vi "Write String Table.vi"(0 "Report Ref In":T1, 1 "Start Row Index":i32, 2 "Start Column Index":i32, 3 "error in (no error)":errorcluster, 4 "Input Range":string[][](array[string])) -> (5 "Report Ref Out":T1, 6 "error out":errorcluster)   [LabVIEW 2013, in "XCel Report Engine.lvlib"]
doc: "Writes a two-dimensional string array to a rectangular range in the active worksheet.\n\nThe top-left destination cell is specified by zero-based row and column coordinates. Coordinate (0, 0) corresponds to cell A1.\n\nThe number of rows and columns is derived from the dimensions of the input array. Values are written in row-major order, and empty strings create empty string cells.\n\nExisting cell values or formulas in the destination range are replaced while the existing formatting of each cell is preserved. The destination range must remain within the Excel worksheet limits."
uses:
  XCel Report Engine.lvlib
  C:/Users/m.santucci/Documents/ChatGPT/LV_REPORT_ENGINE/LV/DotNet/XCelReportEngine.dll
  LV/DotNet/XCelReportEngine.dll
  Controls/Report Ref.ctl
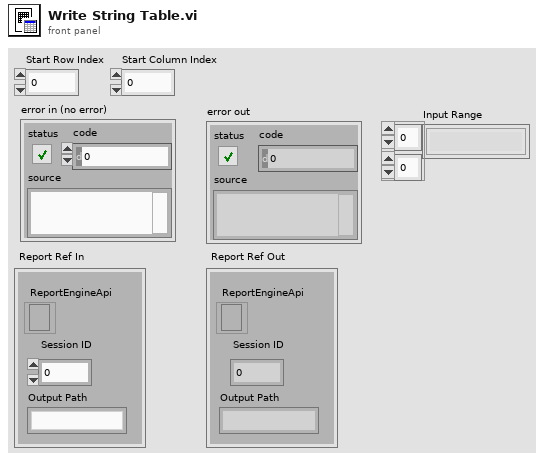
[diagram p1: front panel]
types:
  T1 = typedef "XCel Report Engine.lvlib/Report Ref.ctl" = cluster{"Session ID":i32, "Output Path":string, "ReportEngineApi":refnum<k24>}
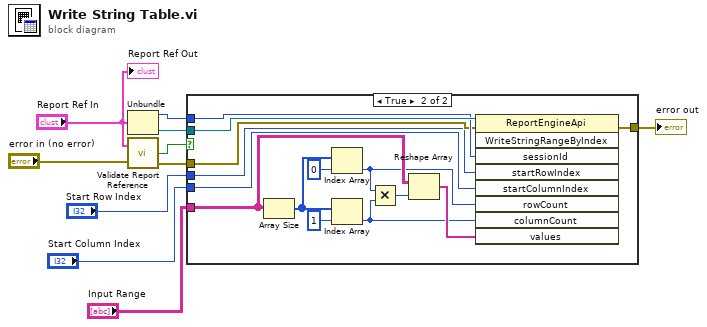
[diagram p0: block diagram]
diagram:
  n1 = Unbundle("Report Ref In") -> ("Session ID"=w8:i32, "ReportEngineApi"=w10:refnum<k24>)  [unwired: 1 out]
  n2 = call "Validate Report Reference.vi"("Report Ref In"="Report Ref In", "error in (no error)"="error in (no error)") -> ("Valid"=w3:bool, "error out"=w4:errorcluster)  [unwired: 1 out]
  n3 = case shown="True" w3 {
    tunnel: w10 -> [_ w25]
    tunnel: [w11 w24] -> w9
    tunnel: w8 -> [_ w23]
    tunnel: "Input Range" -> [_ w22]
    tunnel: w4 -> [w11 w14]
    tunnel: "Start Row Index" -> [_ w13]
    tunnel: "Start Column Index" -> [_ w12]
    frame False {
    }
    frame True {
      n4 = Array Size(array=w22) -> (size(s)=w19:i32[])
      n5 = Index Array(array=w19, index=0) -> (element=w17:i32)
      n6 = Index Array(array=w19, index=1) -> (element=w16:i32)
      n7 = Multiply(x=w17, y=w16) -> (x*y=w15:i32)
      n8 = Reshape Array(w22, w15) -> (w21:string[])
      n9 = invoke class="ReportEngineApi" method="WriteStringRangeByIndex"(reference=w25, error in=w14, "sessionId"=w23, "startRowIndex"=w13, "startColumnIndex"=w12, "rowCount"=w17, "columnCount"=w16, "values"=w21) -> (error out=w24:errorcluster)  [unwired: 1 in, 8 out]
    }
  }
  "error out" <- w9
  "Report Ref Out" <- "Report Ref In"
